vi "Write log to folder.vi"(5 "version":string, 6 "current priority":string, 7 "enabled priority":string, 8 "error in":errorcluster, 9 "resp array":string[](array[string]), 10 "send array":string[](array[string]), 11 "prefix":string) -> (0 "error out":errorcluster, 1 "error":bool, 2 "logged text":string)   [LabVIEW 2018]
panel:
  in  "log path":path
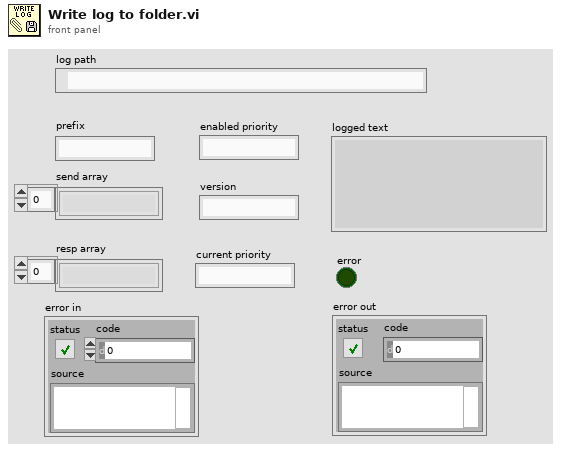
[diagram p1: front panel]
types:
  T1 = enum16{"open", "replace", "create", "open or create", "replace or create", "replace or create with confirmation"}
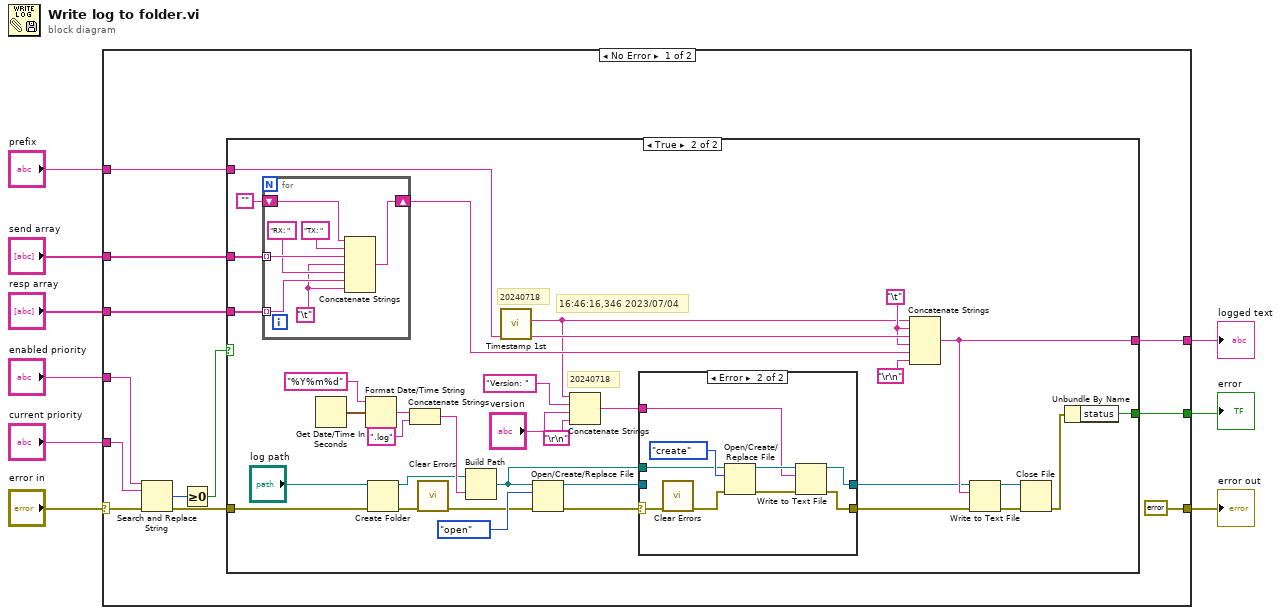
[diagram p0: block diagram]
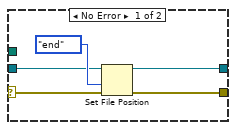
[diagram p3: hidden frame]
diagram:
  n1 = case shown="No Error" "error in" {
    selector: "error in" -> [w14 _]
    tunnel: "enabled priority" -> [w15 _]
    tunnel: [errorcluster {"status"=FALSE, "code"=0, "source"=""} ("error out") _] -> w8
    tunnel: [w21 _] -> w6
    tunnel: "current priority" -> [w12 _]
    tunnel: "resp array" -> [w19 _]
    tunnel: "send array" -> [w18 _]
    tunnel: "prefix" -> [w16 _]
    tunnel: [w17 _] -> w1
    frame No Error {
      n2 = Search and Replace String(input string=w15, search string=w12, error in=w14) -> (number of replacements=w11:i32, error out=w13:errorcluster)  [unwired: 5 in, 2 out]
      n3 = Greater Or Equal To 0?(x=w11) -> (x >= 0?=w10:bool)
      n4 = case shown="True" w10 {
        tunnel: [_ w54] -> w21
        tunnel: w19 -> [_ w53]
        tunnel: w18 -> [_ w52]
        tunnel: [_ w51] -> w17
        tunnel: w16 -> [_ w34]
        tunnel: w13 -> [_ w49]
        frame False {
        }
        frame True {
          w33 = "\t"
          # "20240718"
          # "20240718"
          # "16:46:16,346 2023/07/04"
          n5 = for {
            tunnel: w53 -> [w73] mode=indexing
            tunnel: w52 -> [w75] mode=indexing
            shift-right: [w70] -> w32
            shift-left: "" -> [w71]
            w69 = "\t"
            n6 = Concatenate Strings(w71, "TX: ", w75, w69, "RX: ", w73, w69) -> (w70:string)
          }
          n7 = Get Date/Time In Seconds() -> (seconds since 1Jan1904=w46:timestamp)
          n8 = Format Date/Time String(time format string (%c)="%Y%m%d", seconds (now)=w46) -> (date/time string=w44:string)  [unwired: 1 in]
          n9 = Create Folder(path (use dialog)="log path", error in=w49) -> (created path=w36:path, error out=w38:errorcluster)  [unwired: 1 in, 1 out]
          n10 = Concatenate Strings(w44, ".log" ("string")) -> (w43:string)
          n11 = call <vilib>:"Clear Errors.vi"("error in (no error)"=w38) -> ("error out"=w37:errorcluster)  [unwired: 5 in, 1 out]
          n12 = Build Path(base path=w36, name or relative path=w43) -> (appended path=w27:path)
          n13 = call "Timestamp 1st.vi"() -> ("system timestamp"=w24:string)  [unwired: 11 in]
          n14 = Open/Create/Replace File(file path (use dialog)=w27, error in=w37, operation (0:open)=T1."open") -> (refnum out=w30:refnum<file>, error out=w31:errorcluster)  [unwired: 3 in, 1 out]
          n15 = Concatenate Strings(w24, "Version: " ("string"), "version", "\r\n") -> (w22:string)
          n16 = case shown="Error" w31 {
            selector: w31 -> [w58 w68]
            tunnel: w30 -> [w57 _]
            tunnel: [w56 w61] -> w29
            tunnel: [w55 w62] -> w28
            tunnel: w27 -> [_ w66]
            tunnel: w22 -> [_ w60]
            frame No Error {
              n17 = Set File Position(refnum=w57, from (0:start)=enum16{"start", "end", "current"}."end", error in=w58) -> (refnum out=w56:refnum<file>, error out=w55:errorcluster)  [unwired: 1 in]
            }
            frame Error {
              n18 = call <vilib>:"Clear Errors.vi"("error in (no error)"=w68) -> ("error out"=w65:errorcluster)  [unwired: 5 in, 1 out]
              n19 = Open/Create/Replace File(file path (use dialog)=w66, error in=w65, operation (0:open)=T1."create") -> (refnum out=w63:refnum<file>, error out=w64:errorcluster)  [unwired: 3 in, 1 out]
              n20 = Write to Text File(file (use dialog)=w63, text=w60, error in=w64) -> (refnum out=w61:refnum<file>, error out=w62:errorcluster)  [unwired: 1 in, 1 out]
            }
          }
          n21 = Concatenate Strings(w24, w33, w34, w33, w32, "\r\n") -> (w51:string)
          n22 = Write to Text File(file (use dialog)=w29, text=w51, error in=w28) -> (refnum out=w41:refnum<file>, error out=w40:errorcluster)  [unwired: 1 in, 1 out]
          n23 = Close File(refnum=w41, error in=w40) -> (error out=w39:errorcluster)  [unwired: 1 out]
          n24 = Unbundle By Name(w39) -> ("status"=w54:bool)
        }
      }
    }
    frame Error {
    }
  }
  "error out" <- w8
  "error" <- w6
  "logged text" <- w1
